vi "E10_FormulaNode.vi"() -> ()   [LabVIEW 2026]
panel:
  out "output variable 2":dbl
  out "output variable":dbl[](array[numeric])
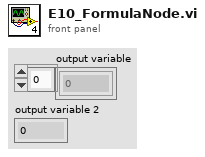
[diagram p1: front panel]
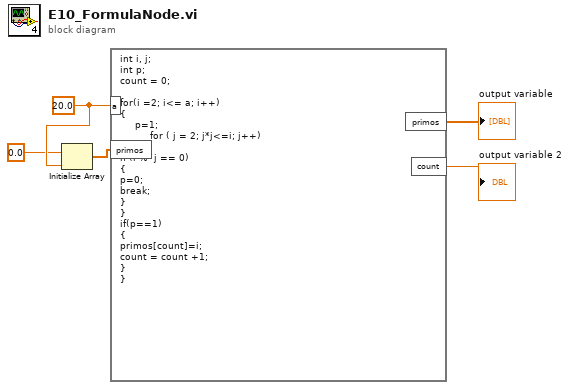
[diagram p0: block diagram]
diagram:
  w5 = 20.0 ("input variable")
  n1 = Initialize Array(0.0 ("element"), w5) -> (w3:dbl[])
  n2 = formula code="int i, j; \nint p;\ncount = 0;\n\nfor(i =2; i<= a; i++)\n{\n     p=1;\n          for ( j = 2; j*j<=i; j++)\n{\nif (i %  j == 0)\n{\np=0;\nbreak;\n}\n}\nif(p==1)\n{\nprimos[count]=i;\ncount = count +1;\n}\n}"("a"=w5, "primos"=w3) -> ("primos"=→"output variable":dbl[], "count"=→"output variable 2":dbl)
